vi "Problem 11 - Largest product in a grid.vi"() -> (3 "Answer":u64)   [LabVIEW 2021, in "Project Euler.lvlib"]
uses:
  Project Euler.lvlib
  Utilities/Numeric Utilities/diagonal direction.ctl
  Utilities/Named Timers/Named Timers.lvlib
  Utilities/Numeric Utilities/Numeric Utilities.lvlib
panel:
  out "User message":string
  out "Array: no. of columns":i32
  out "Array: no. of rows":i32
  out "2D array":i32[][](array[numeric])
  out "Rows":string[](array[string])
  in  "grid":string="08 02 22 97 38 15 00 40 00 75 04 05 07 78 52 12 50 77 91 08\n49 49 99 40 17 81 18 57 60 87 17 40 98 43 69 48 04 56 62 00\n81 49 31 73 55 79 14 29 93 71 40 67 53 88 30 03 49 13 36 65\n52 70 95 23 04 60 11 42 69 24 68 56 01 32 56 71 37 02 36 91\n22 31 16 71 51 67 63 89 41 92 36 54 22 40 40 28 66 33 13 80\n24 47 32 60 99 03 45 02 44 75 33 53 78 36 84 20 35 17 12 50\n32 98 81 28 64 23 67 10 26 38 40 67 59 54 70 66 18 38 64 70\n67 26 20 68 02 62 12 20 95 63 94 39 63 08 40 91 66 49 94 21\n24 55 58 05 66 73 99 26 97 17 78 78 96 83 14 88 34 89 63 72\n21 36 23 09 75 00 76 44 20 45 35 14 00 61 33 97 34 31 33 95\n78 17 53 28 22 75 31 67 15 94 03 80 04 62 16 14 09 53 56 92\n16 39 05 42 96 35 31 47 55 58 88 24 00 17 54 24 36 29 85 57\n86 56 00 48 35 71 89 07 05 44 44 37 44 60 21 58 51 54 17 58\n19 80 81 68 05 94 47 69 28 73 92 13 86 52 17 77 04 89 55 40\n04 52 08 83 97 35 99 16 07 97 57 32 16 26 26 79 33 27 98 66\n88 36 68 87 57 62 20 72 03 46 33 67 46 55 12 32 63 93 53 69\n04 42 16 73 38 25 39 11 24 94 72 18 08 46 29 32 40 62 76 36\n20 69 36 41 72 30 23 88 34 62 99 69 82 67 59 85 74 04 36 16\n20 73 35 29 78 31 90 01 74 31 49 71 48 86 81 16 23 57 05 54\n01 70 54 71 83 51 54 69 16 92 33 48 61 43 52 01 89 19 67 48"
  out "Execution time (ms)":u32
  # "Development\nControls or indicators that are useful for development or testing, but which are not outputs of the VI."
  # "Input\nInputs to the VI"
  # "Output\nOutputs of the VI"
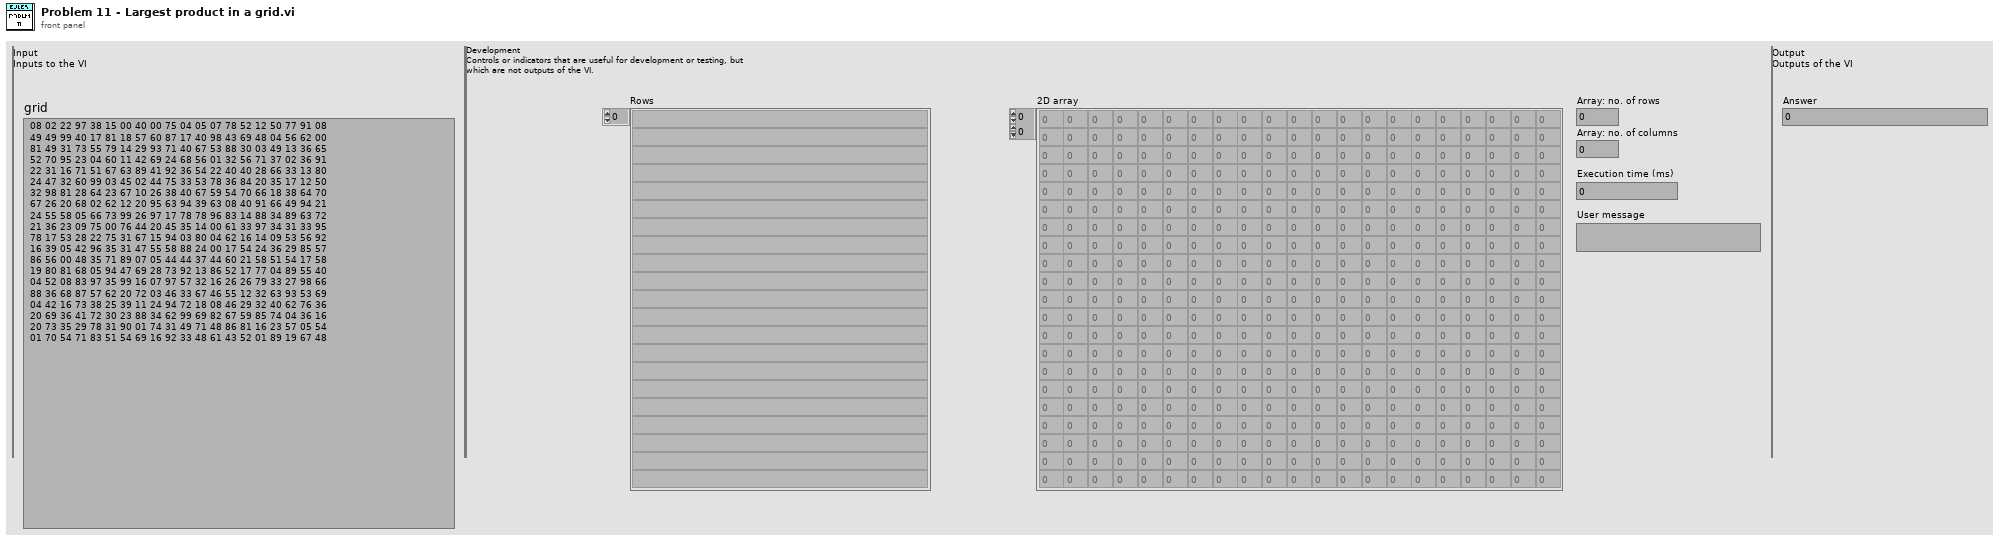
[diagram p1: front panel]
types:
  T1 = typedef "Numeric Utilities.lvlib/diagonal direction.ctl" = enum16{"NW to SE", "SE to NW", "NE to SW", "SW to NE"}
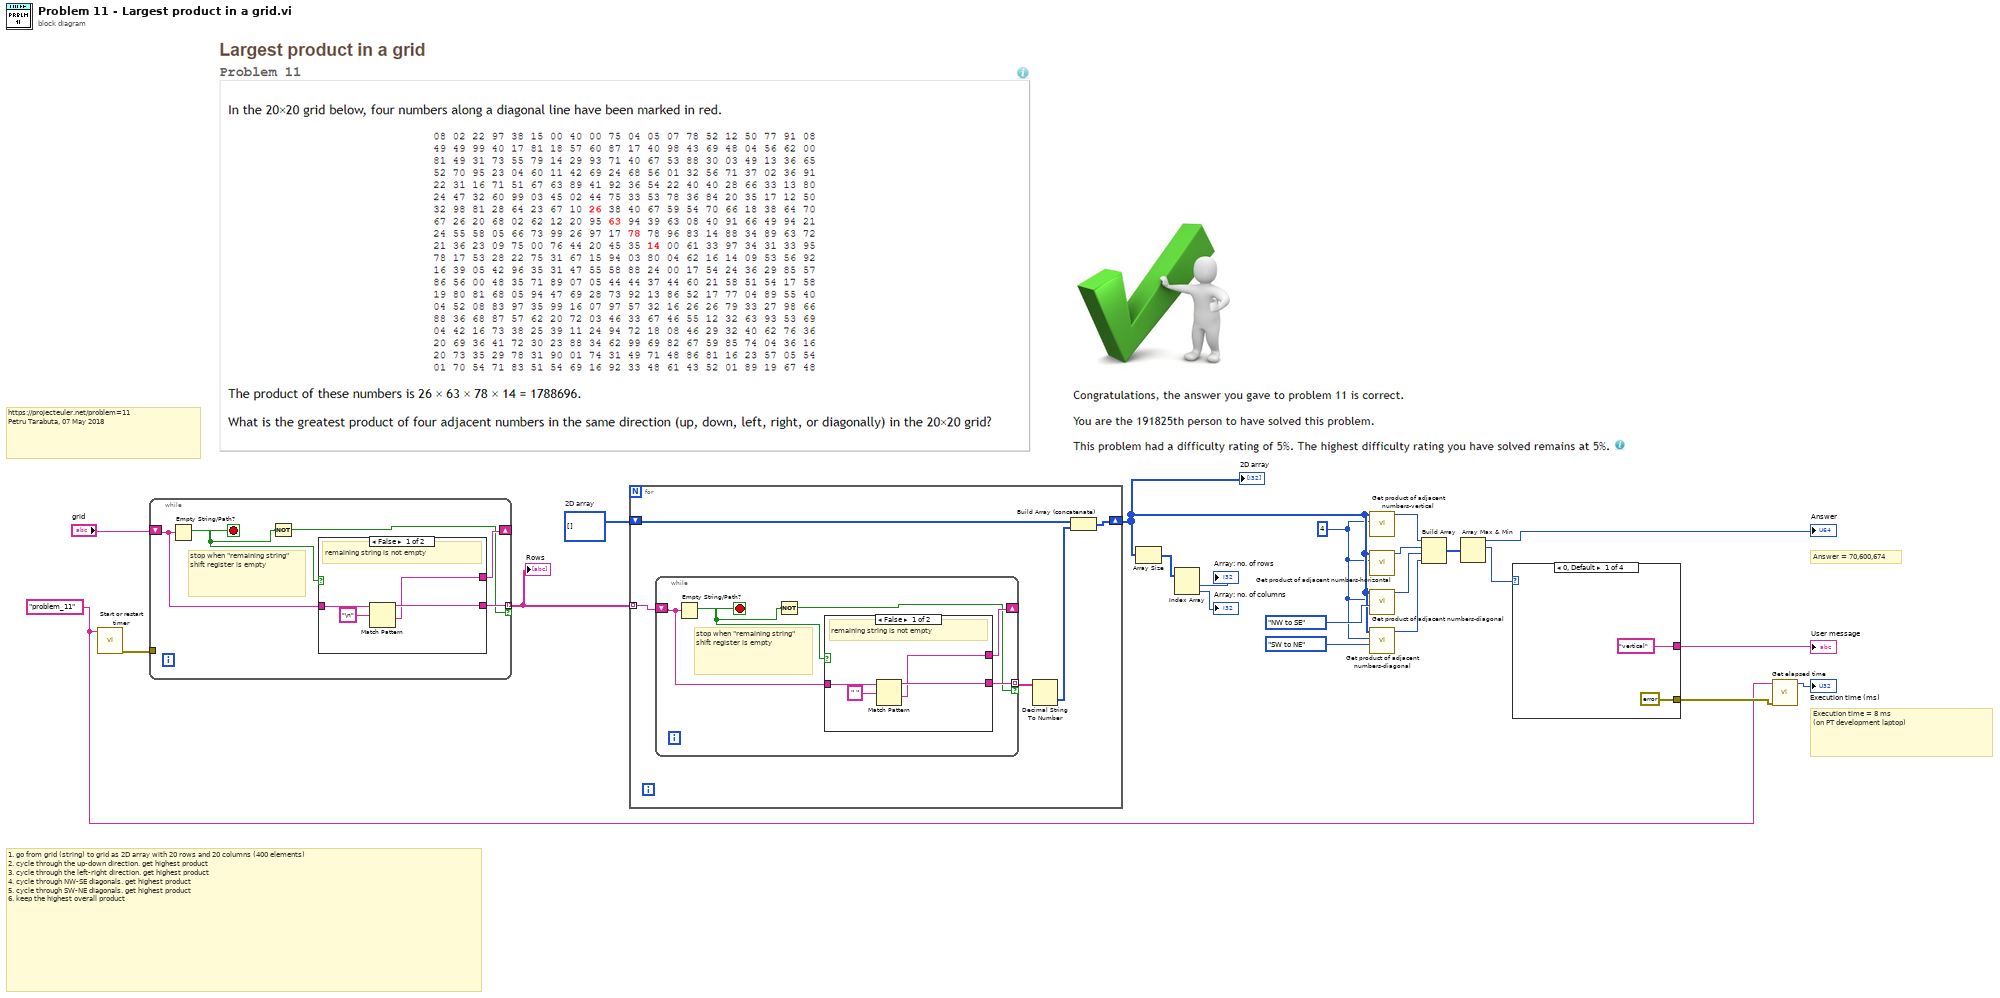
[diagram p0: block diagram]
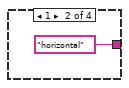
[diagram p2: hidden frame]
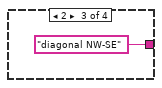
[diagram p3: hidden frame]
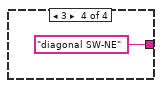
[diagram p4: hidden frame]
diagram:
  w13 = 4 ("How many adjacent numbers? (dflt=4)")
  w19 = i32[][] []  # 2D array
  w1 = "problem_11" ("Counter name (dflt=blank)")
  # "Answer = 70,600,674"
  # "1. go from grid (string) to grid as 2D array with 20 rows and 20 columns (400 elements)\n2. cycle through the up-down direction. get highest product\n3. cycle through the left-right direction. get highest product\n4. cycle through NW-SE diagonals. get highest product\n5. cycle through SW-NE diagonals. get highest product\n6. keep the highest overall product"
  # "Execution time = 8 ms \n(on PT development laptop)"
  # "https://projecteuler.net/problem=11\nPetru Tarabuta, 07 May 2018"
  n1 = call "Start or restart timer.vi"("Timer name"=w1) -> ("error out"=w3:errorcluster)  [unwired: 10 in]
  n2 = while {
    shift-right: [w25] -> _
    shift-left: "grid" -> [w27]
    tunnel: [w26] -> w20 mode=indexing if=w23
    tunnel: w3 -> [_]
    stop <- w24 stop-if-true
    # "stop when \"remaining string\" shift register is empty"
    n3 = Empty String/Path?(string/path=w27) -> (empty?=w24:bool)
    n4 = Not(x=w24) -> (.not. x?=w23:bool)
    n5 = case shown="False" w24 {
      tunnel: w27 -> [w31 w32]
      tunnel: [w29 _] -> w26
      tunnel: [w28 w32] -> w25
      frame False {
        # "remaining string is not empty"
        n6 = Match Pattern(string=w31, regular expression="\n") -> (before substring=w29:string, after substring=w28:string)  [unwired: 1 in, 2 out]
      }
      frame True {
        # "remaining string is empty. do nothing"
      }
    }
  }
  "Rows" <- w20
  n7 = for {
    tunnel: w20 -> [w37] mode=indexing
    shift-right: [w34] -> w14
    shift-left: w19 -> [w35]
    n8 = while {
      shift-right: [w40] -> _
      shift-left: w37 -> [w42]
      tunnel: [w41] -> w36 mode=indexing if=w38
      stop <- w39 stop-if-true
      # "stop when \"remaining string\" shift register is empty"
      n9 = Empty String/Path?(string/path=w42) -> (empty?=w39:bool)
      n10 = Not(x=w39) -> (.not. x?=w38:bool)
      n11 = case shown="False" w39 {
        tunnel: w42 -> [w46 w47]
        tunnel: [w44 _] -> w41
        tunnel: [w43 w47] -> w40
        frame False {
          # "remaining string is not empty"
          n12 = Match Pattern(string=w46, regular expression=" ") -> (before substring=w44:string, after substring=w43:string)  [unwired: 1 in, 2 out]
        }
        frame True {
          # "remaining string is empty. do nothing"
        }
      }
    }
    n13 = Decimal String To Number(string=w36) -> (number=w33:i32[])  [unwired: 2 in, 1 out]
    n14 = Build Array (concatenate)(w35, w33) -> (w34:i32[][])
  }
  "2D array" <- w14
  n15 = Array Size(array=w14) -> (size(s)=w18:i32[])
  n16 = Index Array(array=w18) -> (element #1=→"Array: no. of rows":i32, element #2=→"Array: no. of columns":i32)  [unwired: 2 in]
  n17 = call "Get product of adjacent numbers-vertical.vi"("How many adjacent numbers? (dflt=4)"=w13, "2D array"=w14) -> ("Highest product-vertical direction"=w11:u64)  [unwired: 8 in, 1 out]
  n18 = call "Get product of adjacent numbers-horizontal.vi"("How many adjacent numbers? (dflt=4)"=w13, "2D array"=w14) -> ("Highest product-horizontal direction"=w10:u64)  [unwired: 8 in, 1 out]
  n19 = call "Get product of adjacent numbers-diagonal.vi"("Diagonal direction"=diagonal_direction."NW to SE", "How many adjacent numbers? (dflt=4)"=w13, "2D array"=w14) -> ("Highest product-diagonal direction"=w9:u64)  [unwired: 7 in, 1 out]
  n20 = call "Get product of adjacent numbers-diagonal.vi"("Diagonal direction"=diagonal_direction."SW to NE", "How many adjacent numbers? (dflt=4)"=w13, "2D array"=w14) -> ("Highest product-diagonal direction"=w8:u64)  [unwired: 7 in, 1 out]
  n21 = Build Array(w11, w10, w9, w8) -> (w7:u64[])
  n22 = Array Max & Min(array=w7) -> (max value=→"Answer":u64, max index (indices)=w5:i32)  [unwired: 2 out]
  n23 = case shown="0, Default" w5 {
    tunnel: ["vertical" "horizontal" "diagonal NW-SE" "diagonal SW-NE"] -> w4
    tunnel: [errorcluster {"status"=FALSE, "code"=0, "source"=""} ("error constant") _ _ _] -> w2
    frame 0, Default {
    }
    frame 1 {
    }
    frame 2 {
    }
    frame 3 {
    }
  }
  "User message" <- w4
  n24 = call "Get elapsed time.vi"("error in (no error)"=w2, "Timer name"=w1) -> ("Elapsed time (ms)"=→"Execution time (ms)":u32)  [unwired: 6 in, 3 out]
